vi "Experiment 23.vi"() -> ()   [LabVIEW 2026]
doc: "Experiment 23"
uses:
  <vilib>/AdvancedString/1D String Array to Delimited String (string).vi
  <vilib>/Analysis/baseanly.llb/Mean (DBL).vi
  <vilib>/Analysis/NI_AALBase.lvlib
panel:
  out "No. Of Iterations As Block Of Text (easy to copy into Excel)":string
  out "No. Of Iterations Executed - Loop 10":i32
  out "Output - Loop 10":dbl[](array[numeric]) format="%.3f"
  out "No. Of Iterations Executed - Loop 9":i32
  out "Output - Loop 9":dbl[](array[numeric]) format="%.3f"
  out "No. Of Iterations Executed - Loop 8":i32
  out "Output - Loop 8":dbl[](array[numeric]) format="%.3f"
  out "No. Of Iterations Executed - Loop 7":i32
  out "Output - Loop 7":dbl[](array[numeric]) format="%.3f"
  out "No. Of Iterations Executed - Loop 6":i32
  out "Output - Loop 6":dbl[](array[numeric]) format="%.3f"
  out "No. Of Iterations Executed - Loop 5":i32
  out "Output - Loop 5":dbl[](array[numeric]) format="%.3f"
  out "No. Of Iterations Executed - Loop 4":i32
  out "Output - Loop 4":dbl[](array[numeric]) format="%.3f"
  out "No. Of Iterations Executed - Loop 3":i32
  out "Output - Loop 3":dbl[](array[numeric]) format="%.3f"
  out "Avg. No. Of Iterations Executed - All Loops":dbl format="%.1f"
  out "No. Of Iterations Executed - Loop 2":i32
  out "Output - Loop 2":dbl[](array[numeric]) format="%.3f"
  out "No. Of Iterations Executed - Loop 1":i32
  out "Output - Loop 1":dbl[](array[numeric]) format="%.3f"
  out "Stop VI?":bool
  # "Experiment 23"
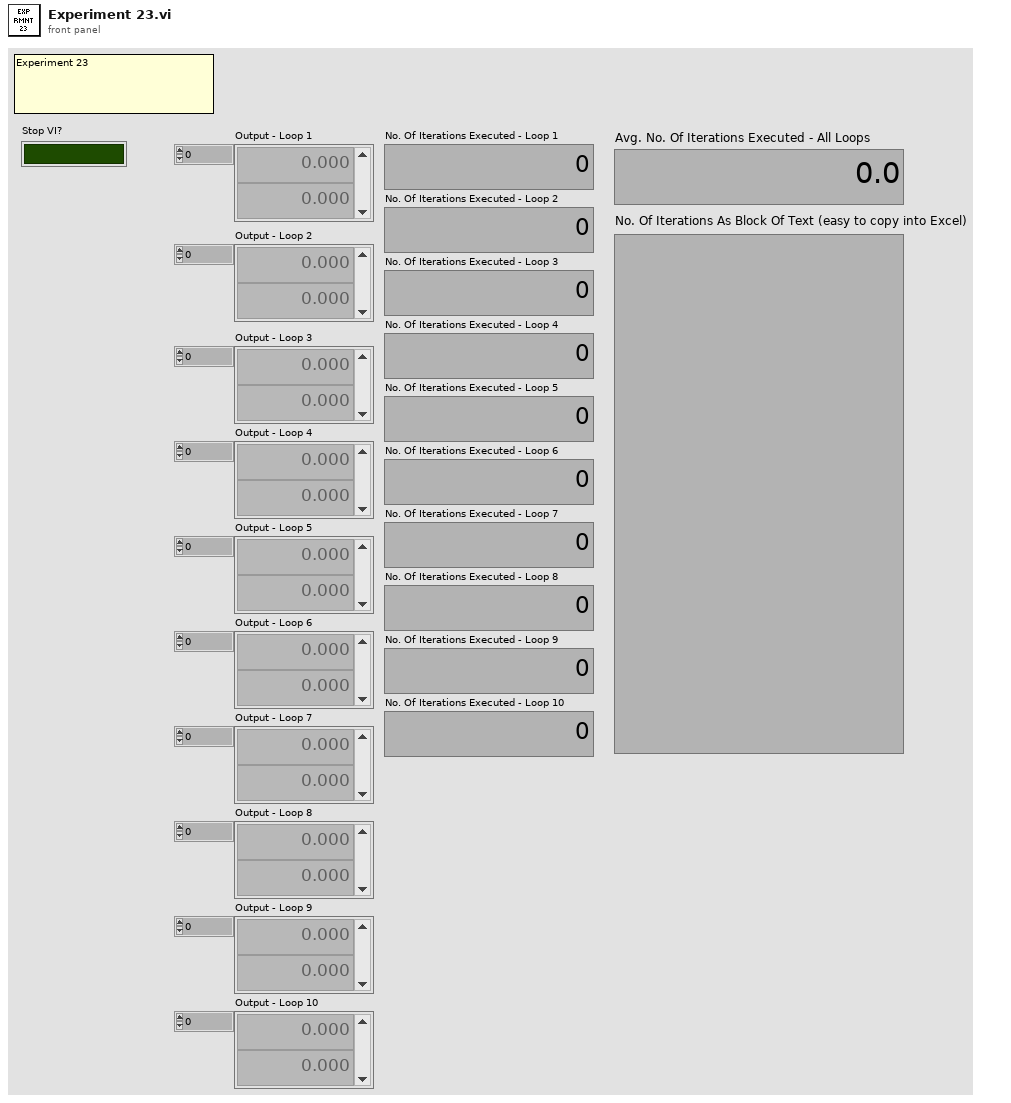
[diagram p1: front panel]
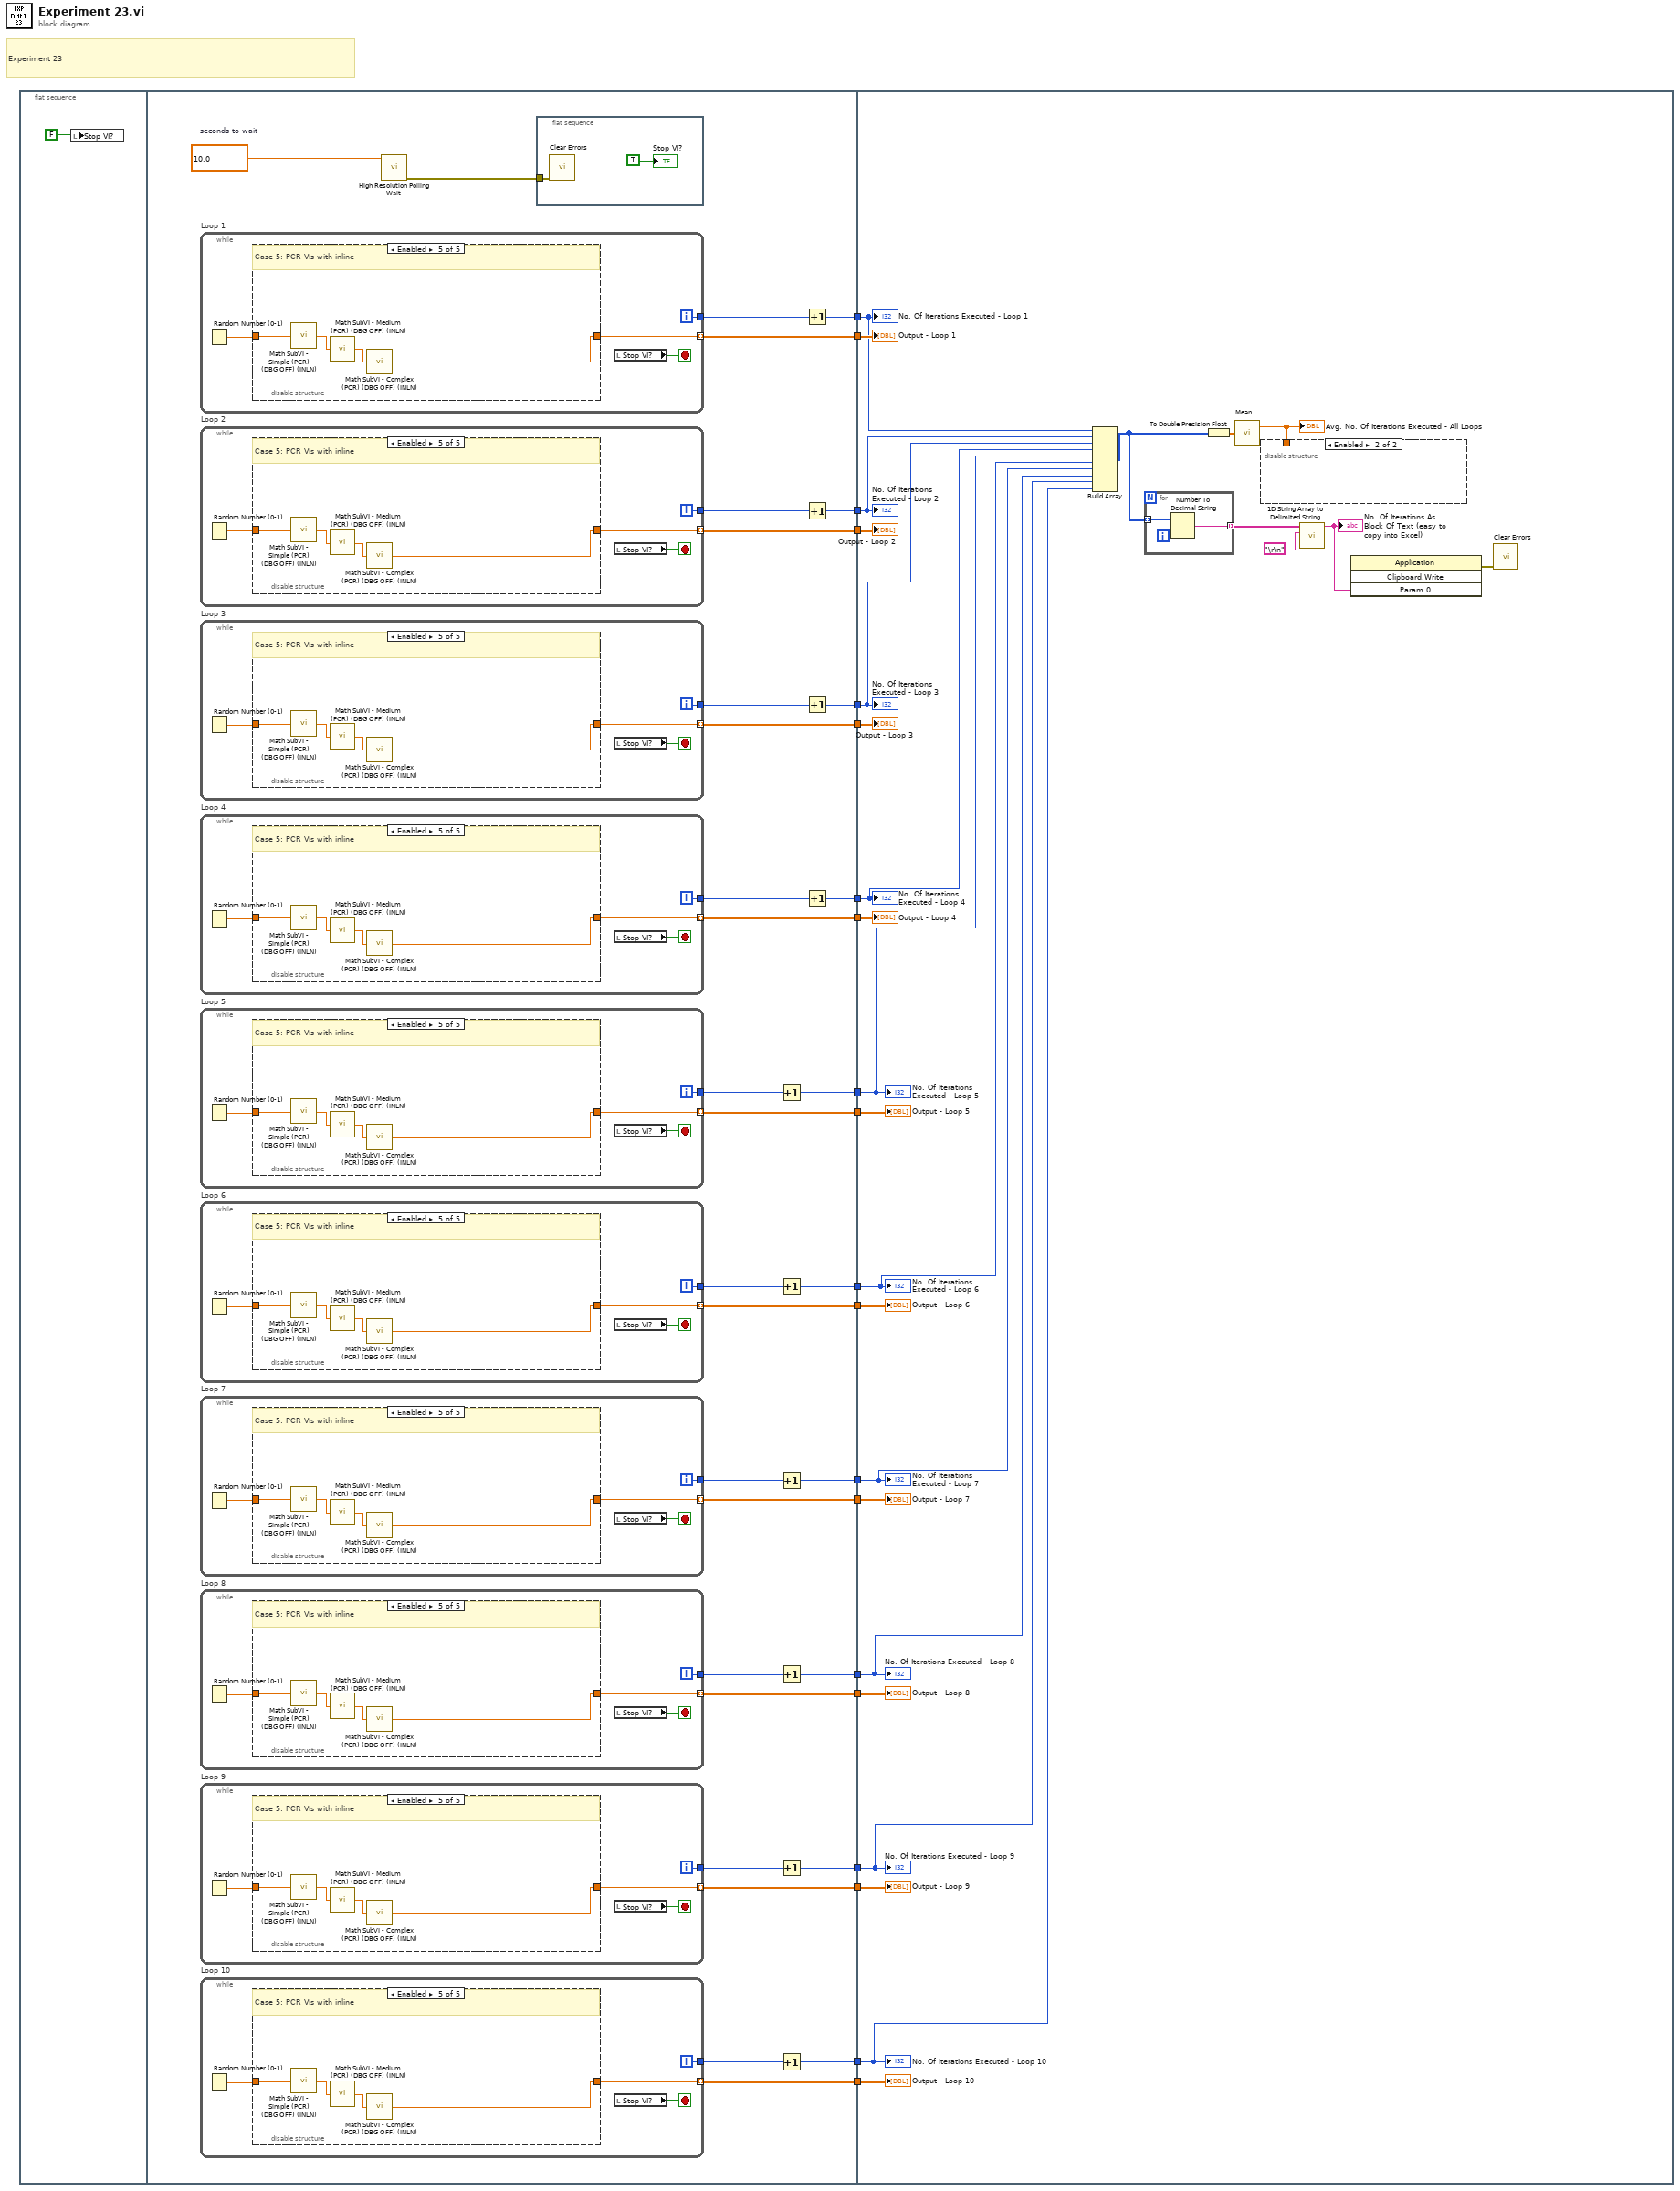
[diagram p0: block diagram]
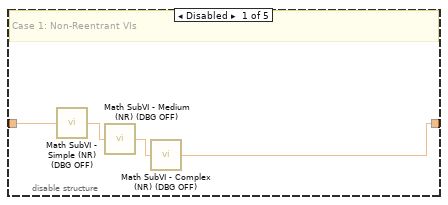
[diagram p2: hidden frame]
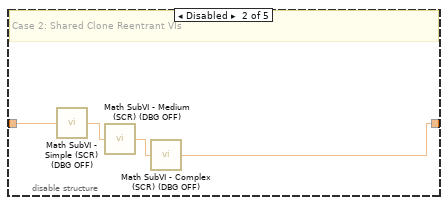
[diagram p3: hidden frame]
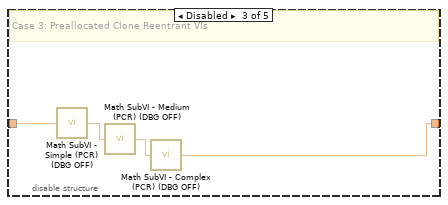
[diagram p4: hidden frame]
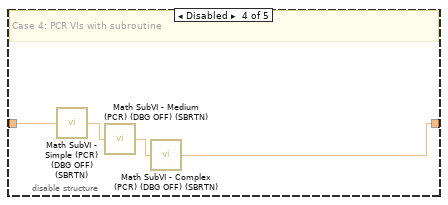
[diagram p5: hidden frame]
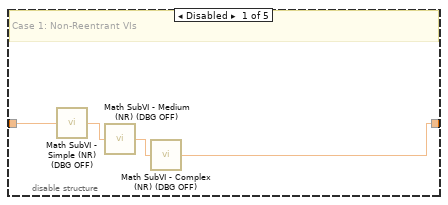
[diagram p6: hidden frame]
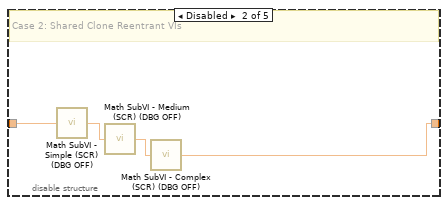
[diagram p7: hidden frame]
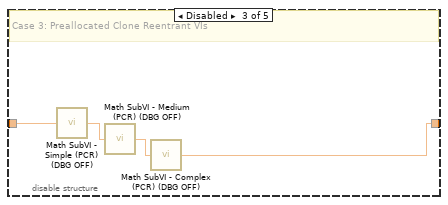
[diagram p8: hidden frame]
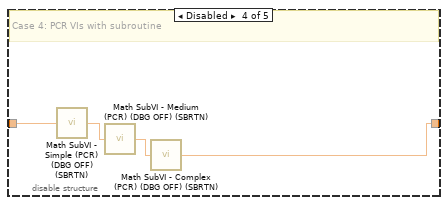
[diagram p9: hidden frame]
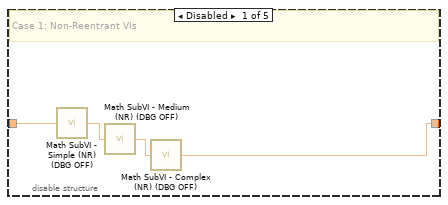
[diagram p10: hidden frame]
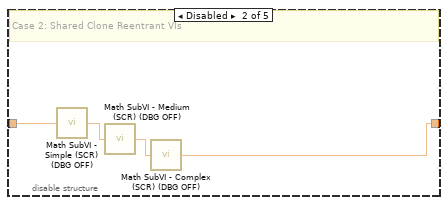
[diagram p11: hidden frame]
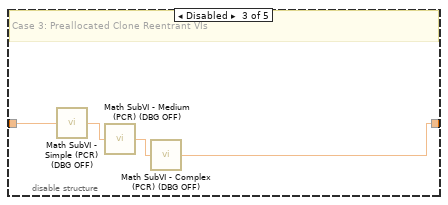
[diagram p12: hidden frame]
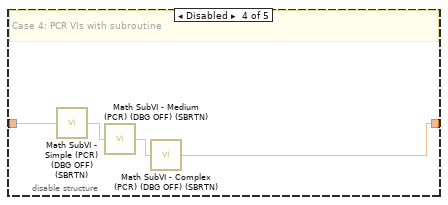
[diagram p13: hidden frame]
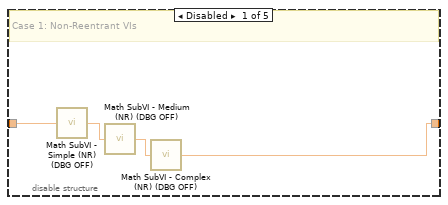
[diagram p14: hidden frame]
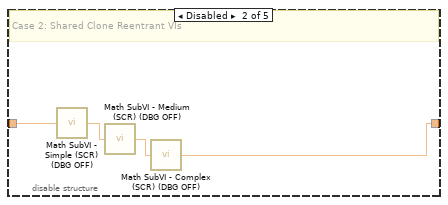
[diagram p15: hidden frame]
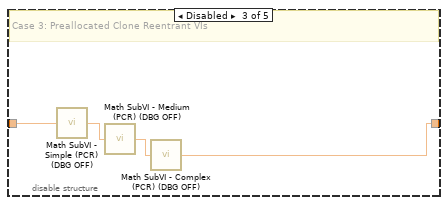
[diagram p16: hidden frame]
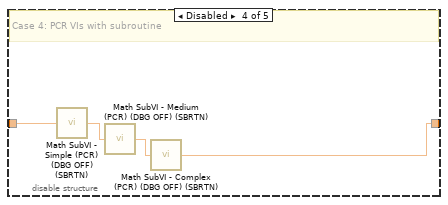
[diagram p17: hidden frame]
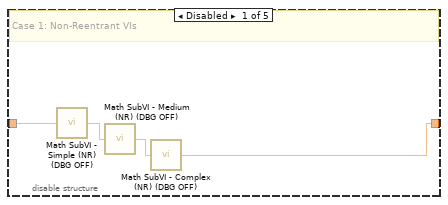
[diagram p18: hidden frame]
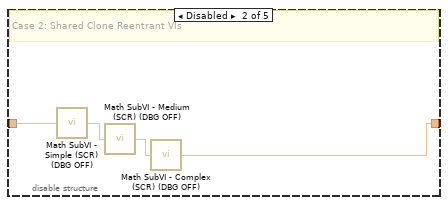
[diagram p19: hidden frame]
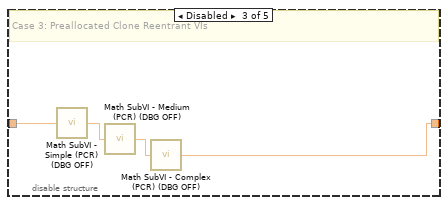
[diagram p20: hidden frame]
diagram:
  # "Experiment 23"
  n1 = flat-sequence {
    tunnel: [w51] -> w20
    tunnel: [w49] -> w19
    tunnel: [w48] -> w18
    tunnel: [w39] -> w17
    tunnel: [w47] -> w16
    tunnel: [w37] -> w15
    tunnel: [w35] -> w14
    tunnel: [w46] -> w13
    tunnel: [w33] -> w12
    tunnel: [w45] -> w11
    tunnel: [w31] -> w10
    tunnel: [w40] -> w9
    tunnel: [w29] -> w8
    tunnel: [w41] -> w7
    tunnel: [w27] -> w6
    tunnel: [w42] -> w5
    tunnel: [w25] -> w4
    tunnel: [w43] -> w3
    tunnel: [w22] -> w2
    tunnel: [w44] -> w1
    tunnel: w20 -> [w322]
    tunnel: w19 -> [w320]
    tunnel: w18 -> [w319]
    tunnel: w17 -> [w321]
    tunnel: w16 -> [w315]
    tunnel: w15 -> [w317]
    tunnel: w14 -> [w316]
    tunnel: w13 -> [w314]
    tunnel: w12 -> [w312]
    tunnel: w11 -> [w306]
    tunnel: w10 -> [w311]
    tunnel: w9 -> [w305]
    tunnel: w8 -> [w310]
    tunnel: w7 -> [w304]
    tunnel: w6 -> [w309]
    tunnel: w5 -> [w303]
    tunnel: w4 -> [w308]
    tunnel: w3 -> [w302]
    tunnel: w2 -> [w307]
    tunnel: w1 -> [w301]
    frame #0 {
      n2 = local write "Stop VI?"(FALSE) -> ()
    }
    frame #1 {
      w53 = 10.0  # seconds to wait
      n3 = while "Loop 1" {
        tunnel: [w271] -> w51 mode=indexing
        tunnel: [w272] -> w50
        i -> [w272]
        stop <- w273 stop-if-true
        n4 = Random Number (0-1)() -> (number: 0 to 1=w270:dbl)
        n5 = disable-structure shown="Enabled" {
          disable-tunnel: w270 -> [w277 w281 w285 w289 w293]
          disable-tunnel: [w276 w280 w284 w288 w292] -> w271
          frame Disabled {
            # "Case 1: Non-Reentrant VIs"
            n6 = call "Math SubVI - Simple (NR) (DBG OFF).vi"("Input"=w277) -> ("Output"=w274:dbl)
            n7 = call "Math SubVI - Medium (NR) (DBG OFF).vi"("Input"=w274) -> ("Output"=w275:dbl)
            n8 = call "Math SubVI - Complex (NR) (DBG OFF).vi"("Input"=w275) -> ("Output"=w276:dbl)
          }
          frame Disabled {
            # "Case 2: Shared Clone Reentrant VIs"
            n9 = call "Math SubVI - Simple (SCR) (DBG OFF).vi"("Input"=w281) -> ("Output"=w278:dbl)
            n10 = call "Math SubVI - Medium (SCR) (DBG OFF).vi"("Input"=w278) -> ("Output"=w279:dbl)
            n11 = call "Math SubVI - Complex (SCR) (DBG OFF).vi"("Input"=w279) -> ("Output"=w280:dbl)
          }
          frame Disabled {
            # "Case 3: Preallocated Clone Reentrant VIs"
            n12 = call "Math SubVI - Simple (PCR) (DBG OFF).vi"("Input"=w285) -> ("Output"=w282:dbl)
            n13 = call "Math SubVI - Medium (PCR) (DBG OFF).vi"("Input"=w282) -> ("Output"=w283:dbl)
            n14 = call "Math SubVI - Complex (PCR) (DBG OFF).vi"("Input"=w283) -> ("Output"=w284:dbl)
          }
          frame Disabled {
            # "Case 4: PCR VIs with subroutine"
            n15 = call "Math SubVI - Simple (PCR) (DBG OFF) (SBRTN).vi"("Input"=w289) -> ("Output"=w286:dbl)
            n16 = call "Math SubVI - Medium (PCR) (DBG OFF) (SBRTN).vi"("Input"=w286) -> ("Output"=w287:dbl)
            n17 = call "Math SubVI - Complex (PCR) (DBG OFF) (SBRTN).vi"("Input"=w287) -> ("Output"=w288:dbl)
          }
          frame Enabled {
            # "Case 5: PCR VIs with inline"
            n18 = call "Math SubVI - Simple (PCR) (DBG OFF) (INLN).vi"("Input"=w293) -> ("Output"=w290:dbl)
            n19 = call "Math SubVI - Medium (PCR) (DBG OFF) (INLN).vi"("Input"=w290) -> ("Output"=w291:dbl)
            n20 = call "Math SubVI - Complex (PCR) (DBG OFF) (INLN).vi"("Input"=w291) -> ("Output"=w292:dbl)
          }
        }
        n21 = local read "Stop VI?"() -> (w273:bool)
      }
      n22 = while "Loop 2" {
        tunnel: [w247] -> w39 mode=indexing
        tunnel: [w248] -> w38
        i -> [w248]
        stop <- w249 stop-if-true
        n23 = Random Number (0-1)() -> (number: 0 to 1=w246:dbl)
        n24 = disable-structure shown="Enabled" {
          disable-tunnel: w246 -> [w253 w257 w261 w265 w269]
          disable-tunnel: [w252 w256 w260 w264 w268] -> w247
          frame Disabled {
            # "Case 1: Non-Reentrant VIs"
            n25 = call "Math SubVI - Simple (NR) (DBG OFF).vi"("Input"=w253) -> ("Output"=w250:dbl)
            n26 = call "Math SubVI - Medium (NR) (DBG OFF).vi"("Input"=w250) -> ("Output"=w251:dbl)
            n27 = call "Math SubVI - Complex (NR) (DBG OFF).vi"("Input"=w251) -> ("Output"=w252:dbl)
          }
          frame Disabled {
            # "Case 2: Shared Clone Reentrant VIs"
            n28 = call "Math SubVI - Simple (SCR) (DBG OFF).vi"("Input"=w257) -> ("Output"=w254:dbl)
            n29 = call "Math SubVI - Medium (SCR) (DBG OFF).vi"("Input"=w254) -> ("Output"=w255:dbl)
            n30 = call "Math SubVI - Complex (SCR) (DBG OFF).vi"("Input"=w255) -> ("Output"=w256:dbl)
          }
          frame Disabled {
            # "Case 3: Preallocated Clone Reentrant VIs"
            n31 = call "Math SubVI - Simple (PCR) (DBG OFF).vi"("Input"=w261) -> ("Output"=w258:dbl)
            n32 = call "Math SubVI - Medium (PCR) (DBG OFF).vi"("Input"=w258) -> ("Output"=w259:dbl)
            n33 = call "Math SubVI - Complex (PCR) (DBG OFF).vi"("Input"=w259) -> ("Output"=w260:dbl)
          }
          frame Disabled {
            # "Case 4: PCR VIs with subroutine"
            n34 = call "Math SubVI - Simple (PCR) (DBG OFF) (SBRTN).vi"("Input"=w265) -> ("Output"=w262:dbl)
            n35 = call "Math SubVI - Medium (PCR) (DBG OFF) (SBRTN).vi"("Input"=w262) -> ("Output"=w263:dbl)
            n36 = call "Math SubVI - Complex (PCR) (DBG OFF) (SBRTN).vi"("Input"=w263) -> ("Output"=w264:dbl)
          }
          frame Enabled {
            # "Case 5: PCR VIs with inline"
            n37 = call "Math SubVI - Simple (PCR) (DBG OFF) (INLN).vi"("Input"=w269) -> ("Output"=w266:dbl)
            n38 = call "Math SubVI - Medium (PCR) (DBG OFF) (INLN).vi"("Input"=w266) -> ("Output"=w267:dbl)
            n39 = call "Math SubVI - Complex (PCR) (DBG OFF) (INLN).vi"("Input"=w267) -> ("Output"=w268:dbl)
          }
        }
        n40 = local read "Stop VI?"() -> (w249:bool)
      }
      n41 = while "Loop 3" {
        tunnel: [w223] -> w37 mode=indexing
        tunnel: [w224] -> w36
        i -> [w224]
        stop <- w225 stop-if-true
        n42 = Random Number (0-1)() -> (number: 0 to 1=w222:dbl)
        n43 = disable-structure shown="Enabled" {
          disable-tunnel: w222 -> [w229 w233 w237 w241 w245]
          disable-tunnel: [w228 w232 w236 w240 w244] -> w223
          frame Disabled {
            # "Case 1: Non-Reentrant VIs"
            n44 = call "Math SubVI - Simple (NR) (DBG OFF).vi"("Input"=w229) -> ("Output"=w226:dbl)
            n45 = call "Math SubVI - Medium (NR) (DBG OFF).vi"("Input"=w226) -> ("Output"=w227:dbl)
            n46 = call "Math SubVI - Complex (NR) (DBG OFF).vi"("Input"=w227) -> ("Output"=w228:dbl)
          }
          frame Disabled {
            # "Case 2: Shared Clone Reentrant VIs"
            n47 = call "Math SubVI - Simple (SCR) (DBG OFF).vi"("Input"=w233) -> ("Output"=w230:dbl)
            n48 = call "Math SubVI - Medium (SCR) (DBG OFF).vi"("Input"=w230) -> ("Output"=w231:dbl)
            n49 = call "Math SubVI - Complex (SCR) (DBG OFF).vi"("Input"=w231) -> ("Output"=w232:dbl)
          }
          frame Disabled {
            # "Case 3: Preallocated Clone Reentrant VIs"
            n50 = call "Math SubVI - Simple (PCR) (DBG OFF).vi"("Input"=w237) -> ("Output"=w234:dbl)
            n51 = call "Math SubVI - Medium (PCR) (DBG OFF).vi"("Input"=w234) -> ("Output"=w235:dbl)
            n52 = call "Math SubVI - Complex (PCR) (DBG OFF).vi"("Input"=w235) -> ("Output"=w236:dbl)
          }
          frame Disabled {
            # "Case 4: PCR VIs with subroutine"
            n53 = call "Math SubVI - Simple (PCR) (DBG OFF) (SBRTN).vi"("Input"=w241) -> ("Output"=w238:dbl)
            n54 = call "Math SubVI - Medium (PCR) (DBG OFF) (SBRTN).vi"("Input"=w238) -> ("Output"=w239:dbl)
            n55 = call "Math SubVI - Complex (PCR) (DBG OFF) (SBRTN).vi"("Input"=w239) -> ("Output"=w240:dbl)
          }
          frame Enabled {
            # "Case 5: PCR VIs with inline"
            n56 = call "Math SubVI - Simple (PCR) (DBG OFF) (INLN).vi"("Input"=w245) -> ("Output"=w242:dbl)
            n57 = call "Math SubVI - Medium (PCR) (DBG OFF) (INLN).vi"("Input"=w242) -> ("Output"=w243:dbl)
            n58 = call "Math SubVI - Complex (PCR) (DBG OFF) (INLN).vi"("Input"=w243) -> ("Output"=w244:dbl)
          }
        }
        n59 = local read "Stop VI?"() -> (w225:bool)
      }
      n60 = while "Loop 4" {
        tunnel: [w199] -> w35 mode=indexing
        tunnel: [w200] -> w34
        i -> [w200]
        stop <- w201 stop-if-true
        n61 = Random Number (0-1)() -> (number: 0 to 1=w198:dbl)
        n62 = disable-structure shown="Enabled" {
          disable-tunnel: w198 -> [w205 w209 w213 w217 w221]
          disable-tunnel: [w204 w208 w212 w216 w220] -> w199
          frame Disabled {
            # "Case 1: Non-Reentrant VIs"
            n63 = call "Math SubVI - Simple (NR) (DBG OFF).vi"("Input"=w205) -> ("Output"=w202:dbl)
            n64 = call "Math SubVI - Medium (NR) (DBG OFF).vi"("Input"=w202) -> ("Output"=w203:dbl)
            n65 = call "Math SubVI - Complex (NR) (DBG OFF).vi"("Input"=w203) -> ("Output"=w204:dbl)
          }
          frame Disabled {
            # "Case 2: Shared Clone Reentrant VIs"
            n66 = call "Math SubVI - Simple (SCR) (DBG OFF).vi"("Input"=w209) -> ("Output"=w206:dbl)
            n67 = call "Math SubVI - Medium (SCR) (DBG OFF).vi"("Input"=w206) -> ("Output"=w207:dbl)
            n68 = call "Math SubVI - Complex (SCR) (DBG OFF).vi"("Input"=w207) -> ("Output"=w208:dbl)
          }
          frame Disabled {
            # "Case 3: Preallocated Clone Reentrant VIs"
            n69 = call "Math SubVI - Simple (PCR) (DBG OFF).vi"("Input"=w213) -> ("Output"=w210:dbl)
            n70 = call "Math SubVI - Medium (PCR) (DBG OFF).vi"("Input"=w210) -> ("Output"=w211:dbl)
            n71 = call "Math SubVI - Complex (PCR) (DBG OFF).vi"("Input"=w211) -> ("Output"=w212:dbl)
          }
          frame Disabled {
            # "Case 4: PCR VIs with subroutine"
            n72 = call "Math SubVI - Simple (PCR) (DBG OFF) (SBRTN).vi"("Input"=w217) -> ("Output"=w214:dbl)
            n73 = call "Math SubVI - Medium (PCR) (DBG OFF) (SBRTN).vi"("Input"=w214) -> ("Output"=w215:dbl)
            n74 = call "Math SubVI - Complex (PCR) (DBG OFF) (SBRTN).vi"("Input"=w215) -> ("Output"=w216:dbl)
          }
          frame Enabled {
            # "Case 5: PCR VIs with inline"
            n75 = call "Math SubVI - Simple (PCR) (DBG OFF) (INLN).vi"("Input"=w221) -> ("Output"=w218:dbl)
            n76 = call "Math SubVI - Medium (PCR) (DBG OFF) (INLN).vi"("Input"=w218) -> ("Output"=w219:dbl)
            n77 = call "Math SubVI - Complex (PCR) (DBG OFF) (INLN).vi"("Input"=w219) -> ("Output"=w220:dbl)
          }
        }
        n78 = local read "Stop VI?"() -> (w201:bool)
      }
      n79 = while "Loop 5" {
        tunnel: [w175] -> w33 mode=indexing
        tunnel: [w176] -> w32
        i -> [w176]
        stop <- w177 stop-if-true
        n80 = Random Number (0-1)() -> (number: 0 to 1=w174:dbl)
        n81 = disable-structure shown="Enabled" {
          disable-tunnel: w174 -> [w181 w185 w189 w193 w197]
          disable-tunnel: [w180 w184 w188 w192 w196] -> w175
          frame Disabled {
            # "Case 1: Non-Reentrant VIs"
            n82 = call "Math SubVI - Simple (NR) (DBG OFF).vi"("Input"=w181) -> ("Output"=w178:dbl)
            n83 = call "Math SubVI - Medium (NR) (DBG OFF).vi"("Input"=w178) -> ("Output"=w179:dbl)
            n84 = call "Math SubVI - Complex (NR) (DBG OFF).vi"("Input"=w179) -> ("Output"=w180:dbl)
          }
          frame Disabled {
            # "Case 2: Shared Clone Reentrant VIs"
            n85 = call "Math SubVI - Simple (SCR) (DBG OFF).vi"("Input"=w185) -> ("Output"=w182:dbl)
            n86 = call "Math SubVI - Medium (SCR) (DBG OFF).vi"("Input"=w182) -> ("Output"=w183:dbl)
            n87 = call "Math SubVI - Complex (SCR) (DBG OFF).vi"("Input"=w183) -> ("Output"=w184:dbl)
          }
          frame Disabled {
            # "Case 3: Preallocated Clone Reentrant VIs"
            n88 = call "Math SubVI - Simple (PCR) (DBG OFF).vi"("Input"=w189) -> ("Output"=w186:dbl)
            n89 = call "Math SubVI - Medium (PCR) (DBG OFF).vi"("Input"=w186) -> ("Output"=w187:dbl)
            n90 = call "Math SubVI - Complex (PCR) (DBG OFF).vi"("Input"=w187) -> ("Output"=w188:dbl)
          }
          frame Disabled {
            # "Case 4: PCR VIs with subroutine"
            n91 = call "Math SubVI - Simple (PCR) (DBG OFF) (SBRTN).vi"("Input"=w193) -> ("Output"=w190:dbl)
            n92 = call "Math SubVI - Medium (PCR) (DBG OFF) (SBRTN).vi"("Input"=w190) -> ("Output"=w191:dbl)
            n93 = call "Math SubVI - Complex (PCR) (DBG OFF) (SBRTN).vi"("Input"=w191) -> ("Output"=w192:dbl)
          }
          frame Enabled {
            # "Case 5: PCR VIs with inline"
            n94 = call "Math SubVI - Simple (PCR) (DBG OFF) (INLN).vi"("Input"=w197) -> ("Output"=w194:dbl)
            n95 = call "Math SubVI - Medium (PCR) (DBG OFF) (INLN).vi"("Input"=w194) -> ("Output"=w195:dbl)
            n96 = call "Math SubVI - Complex (PCR) (DBG OFF) (INLN).vi"("Input"=w195) -> ("Output"=w196:dbl)
          }
        }
        n97 = local read "Stop VI?"() -> (w177:bool)
      }
      n98 = while "Loop 6" {
        tunnel: [w151] -> w31 mode=indexing
        tunnel: [w152] -> w30
        i -> [w152]
        stop <- w153 stop-if-true
        n99 = Random Number (0-1)() -> (number: 0 to 1=w150:dbl)
        n100 = disable-structure shown="Enabled" {
          disable-tunnel: w150 -> [w157 w161 w165 w169 w173]
          disable-tunnel: [w156 w160 w164 w168 w172] -> w151
          frame Disabled {
            # "Case 1: Non-Reentrant VIs"
            n101 = call "Math SubVI - Simple (NR) (DBG OFF).vi"("Input"=w157) -> ("Output"=w154:dbl)
            n102 = call "Math SubVI - Medium (NR) (DBG OFF).vi"("Input"=w154) -> ("Output"=w155:dbl)
            n103 = call "Math SubVI - Complex (NR) (DBG OFF).vi"("Input"=w155) -> ("Output"=w156:dbl)
          }
          frame Disabled {
            # "Case 2: Shared Clone Reentrant VIs"
            n104 = call "Math SubVI - Simple (SCR) (DBG OFF).vi"("Input"=w161) -> ("Output"=w158:dbl)
            n105 = call "Math SubVI - Medium (SCR) (DBG OFF).vi"("Input"=w158) -> ("Output"=w159:dbl)
            n106 = call "Math SubVI - Complex (SCR) (DBG OFF).vi"("Input"=w159) -> ("Output"=w160:dbl)
          }
          frame Disabled {
            # "Case 3: Preallocated Clone Reentrant VIs"
            n107 = call "Math SubVI - Simple (PCR) (DBG OFF).vi"("Input"=w165) -> ("Output"=w162:dbl)
            n108 = call "Math SubVI - Medium (PCR) (DBG OFF).vi"("Input"=w162) -> ("Output"=w163:dbl)
            n109 = call "Math SubVI - Complex (PCR) (DBG OFF).vi"("Input"=w163) -> ("Output"=w164:dbl)
          }
          frame Disabled {
            # "Case 4: PCR VIs with subroutine"
            n110 = call "Math SubVI - Simple (PCR) (DBG OFF) (SBRTN).vi"("Input"=w169) -> ("Output"=w166:dbl)
            n111 = call "Math SubVI - Medium (PCR) (DBG OFF) (SBRTN).vi"("Input"=w166) -> ("Output"=w167:dbl)
            n112 = call "Math SubVI - Complex (PCR) (DBG OFF) (SBRTN).vi"("Input"=w167) -> ("Output"=w168:dbl)
          }
          frame Enabled {
            # "Case 5: PCR VIs with inline"
            n113 = call "Math SubVI - Simple (PCR) (DBG OFF) (INLN).vi"("Input"=w173) -> ("Output"=w170:dbl)
            n114 = call "Math SubVI - Medium (PCR) (DBG OFF) (INLN).vi"("Input"=w170) -> ("Output"=w171:dbl)
            n115 = call "Math SubVI - Complex (PCR) (DBG OFF) (INLN).vi"("Input"=w171) -> ("Output"=w172:dbl)
          }
        }
        n116 = local read "Stop VI?"() -> (w153:bool)
      }
      n117 = while "Loop 7" {
        tunnel: [w127] -> w29 mode=indexing
        tunnel: [w128] -> w28
        i -> [w128]
        stop <- w129 stop-if-true
        n118 = Random Number (0-1)() -> (number: 0 to 1=w126:dbl)
        n119 = disable-structure shown="Enabled" {
          disable-tunnel: w126 -> [w133 w137 w141 w145 w149]
          disable-tunnel: [w132 w136 w140 w144 w148] -> w127
          frame Disabled {
            # "Case 1: Non-Reentrant VIs"
            n120 = call "Math SubVI - Simple (NR) (DBG OFF).vi"("Input"=w133) -> ("Output"=w130:dbl)
            n121 = call "Math SubVI - Medium (NR) (DBG OFF).vi"("Input"=w130) -> ("Output"=w131:dbl)
            n122 = call "Math SubVI - Complex (NR) (DBG OFF).vi"("Input"=w131) -> ("Output"=w132:dbl)
          }
          frame Disabled {
            # "Case 2: Shared Clone Reentrant VIs"
            n123 = call "Math SubVI - Simple (SCR) (DBG OFF).vi"("Input"=w137) -> ("Output"=w134:dbl)
            n124 = call "Math SubVI - Medium (SCR) (DBG OFF).vi"("Input"=w134) -> ("Output"=w135:dbl)
            n125 = call "Math SubVI - Complex (SCR) (DBG OFF).vi"("Input"=w135) -> ("Output"=w136:dbl)
          }
          frame Disabled {
            # "Case 3: Preallocated Clone Reentrant VIs"
            n126 = call "Math SubVI - Simple (PCR) (DBG OFF).vi"("Input"=w141) -> ("Output"=w138:dbl)
            n127 = call "Math SubVI - Medium (PCR) (DBG OFF).vi"("Input"=w138) -> ("Output"=w139:dbl)
            n128 = call "Math SubVI - Complex (PCR) (DBG OFF).vi"("Input"=w139) -> ("Output"=w140:dbl)
          }
          frame Disabled {
            # "Case 4: PCR VIs with subroutine"
            n129 = call "Math SubVI - Simple (PCR) (DBG OFF) (SBRTN).vi"("Input"=w145) -> ("Output"=w142:dbl)
            n130 = call "Math SubVI - Medium (PCR) (DBG OFF) (SBRTN).vi"("Input"=w142) -> ("Output"=w143:dbl)
            n131 = call "Math SubVI - Complex (PCR) (DBG OFF) (SBRTN).vi"("Input"=w143) -> ("Output"=w144:dbl)
          }
          frame Enabled {
            # "Case 5: PCR VIs with inline"
            n132 = call "Math SubVI - Simple (PCR) (DBG OFF) (INLN).vi"("Input"=w149) -> ("Output"=w146:dbl)
            n133 = call "Math SubVI - Medium (PCR) (DBG OFF) (INLN).vi"("Input"=w146) -> ("Output"=w147:dbl)
            n134 = call "Math SubVI - Complex (PCR) (DBG OFF) (INLN).vi"("Input"=w147) -> ("Output"=w148:dbl)
          }
        }
        n135 = local read "Stop VI?"() -> (w129:bool)
      }
      n136 = while "Loop 8" {
        tunnel: [w103] -> w27 mode=indexing
        tunnel: [w104] -> w26
        i -> [w104]
        stop <- w105 stop-if-true
        n137 = Random Number (0-1)() -> (number: 0 to 1=w102:dbl)
        n138 = disable-structure shown="Enabled" {
          disable-tunnel: w102 -> [w109 w113 w117 w121 w125]
          disable-tunnel: [w108 w112 w116 w120 w124] -> w103
          frame Disabled {
            # "Case 1: Non-Reentrant VIs"
            n139 = call "Math SubVI - Simple (NR) (DBG OFF).vi"("Input"=w109) -> ("Output"=w106:dbl)
            n140 = call "Math SubVI - Medium (NR) (DBG OFF).vi"("Input"=w106) -> ("Output"=w107:dbl)
            n141 = call "Math SubVI - Complex (NR) (DBG OFF).vi"("Input"=w107) -> ("Output"=w108:dbl)
          }
          frame Disabled {
            # "Case 2: Shared Clone Reentrant VIs"
            n142 = call "Math SubVI - Simple (SCR) (DBG OFF).vi"("Input"=w113) -> ("Output"=w110:dbl)
            n143 = call "Math SubVI - Medium (SCR) (DBG OFF).vi"("Input"=w110) -> ("Output"=w111:dbl)
            n144 = call "Math SubVI - Complex (SCR) (DBG OFF).vi"("Input"=w111) -> ("Output"=w112:dbl)
          }
          frame Disabled {
            # "Case 3: Preallocated Clone Reentrant VIs"
            n145 = call "Math SubVI - Simple (PCR) (DBG OFF).vi"("Input"=w117) -> ("Output"=w114:dbl)
            n146 = call "Math SubVI - Medium (PCR) (DBG OFF).vi"("Input"=w114) -> ("Output"=w115:dbl)
            n147 = call "Math SubVI - Complex (PCR) (DBG OFF).vi"("Input"=w115) -> ("Output"=w116:dbl)
          }
          frame Disabled {
            # "Case 4: PCR VIs with subroutine"
            n148 = call "Math SubVI - Simple (PCR) (DBG OFF) (SBRTN).vi"("Input"=w121) -> ("Output"=w118:dbl)
            n149 = call "Math SubVI - Medium (PCR) (DBG OFF) (SBRTN).vi"("Input"=w118) -> ("Output"=w119:dbl)
            n150 = call "Math SubVI - Complex (PCR) (DBG OFF) (SBRTN).vi"("Input"=w119) -> ("Output"=w120:dbl)
          }
          frame Enabled {
            # "Case 5: PCR VIs with inline"
            n151 = call "Math SubVI - Simple (PCR) (DBG OFF) (INLN).vi"("Input"=w125) -> ("Output"=w122:dbl)
            n152 = call "Math SubVI - Medium (PCR) (DBG OFF) (INLN).vi"("Input"=w122) -> ("Output"=w123:dbl)
            n153 = call "Math SubVI - Complex (PCR) (DBG OFF) (INLN).vi"("Input"=w123) -> ("Output"=w124:dbl)
          }
        }
        n154 = local read "Stop VI?"() -> (w105:bool)
      }
      n155 = while "Loop 9" {
        tunnel: [w79] -> w25 mode=indexing
        tunnel: [w80] -> w24
        i -> [w80]
        stop <- w81 stop-if-true
        n156 = Random Number (0-1)() -> (number: 0 to 1=w78:dbl)
        n157 = disable-structure shown="Enabled" {
          disable-tunnel: w78 -> [w85 w89 w93 w97 w101]
          disable-tunnel: [w84 w88 w92 w96 w100] -> w79
          frame Disabled {
            # "Case 1: Non-Reentrant VIs"
            n158 = call "Math SubVI - Simple (NR) (DBG OFF).vi"("Input"=w85) -> ("Output"=w82:dbl)
            n159 = call "Math SubVI - Medium (NR) (DBG OFF).vi"("Input"=w82) -> ("Output"=w83:dbl)
            n160 = call "Math SubVI - Complex (NR) (DBG OFF).vi"("Input"=w83) -> ("Output"=w84:dbl)
          }
          frame Disabled {
            # "Case 2: Shared Clone Reentrant VIs"
            n161 = call "Math SubVI - Simple (SCR) (DBG OFF).vi"("Input"=w89) -> ("Output"=w86:dbl)
            n162 = call "Math SubVI - Medium (SCR) (DBG OFF).vi"("Input"=w86) -> ("Output"=w87:dbl)
            n163 = call "Math SubVI - Complex (SCR) (DBG OFF).vi"("Input"=w87) -> ("Output"=w88:dbl)
          }
          frame Disabled {
            # "Case 3: Preallocated Clone Reentrant VIs"
            n164 = call "Math SubVI - Simple (PCR) (DBG OFF).vi"("Input"=w93) -> ("Output"=w90:dbl)
            n165 = call "Math SubVI - Medium (PCR) (DBG OFF).vi"("Input"=w90) -> ("Output"=w91:dbl)
            n166 = call "Math SubVI - Complex (PCR) (DBG OFF).vi"("Input"=w91) -> ("Output"=w92:dbl)
          }
          frame Disabled {
            # "Case 4: PCR VIs with subroutine"
            n167 = call "Math SubVI - Simple (PCR) (DBG OFF) (SBRTN).vi"("Input"=w97) -> ("Output"=w94:dbl)
            n168 = call "Math SubVI - Medium (PCR) (DBG OFF) (SBRTN).vi"("Input"=w94) -> ("Output"=w95:dbl)
            n169 = call "Math SubVI - Complex (PCR) (DBG OFF) (SBRTN).vi"("Input"=w95) -> ("Output"=w96:dbl)
          }
          frame Enabled {
            # "Case 5: PCR VIs with inline"
            n170 = call "Math SubVI - Simple (PCR) (DBG OFF) (INLN).vi"("Input"=w101) -> ("Output"=w98:dbl)
            n171 = call "Math SubVI - Medium (PCR) (DBG OFF) (INLN).vi"("Input"=w98) -> ("Output"=w99:dbl)
            n172 = call "Math SubVI - Complex (PCR) (DBG OFF) (INLN).vi"("Input"=w99) -> ("Output"=w100:dbl)
          }
        }
        n173 = local read "Stop VI?"() -> (w81:bool)
      }
      n174 = while "Loop 10" {
        tunnel: [w55] -> w22 mode=indexing
        tunnel: [w56] -> w23
        i -> [w56]
        stop <- w57 stop-if-true
        n175 = Random Number (0-1)() -> (number: 0 to 1=w54:dbl)
        n176 = disable-structure shown="Enabled" {
          disable-tunnel: w54 -> [w61 w65 w69 w73 w77]
          disable-tunnel: [w60 w64 w68 w72 w76] -> w55
          frame Disabled {
            # "Case 1: Non-Reentrant VIs"
            n177 = call "Math SubVI - Simple (NR) (DBG OFF).vi"("Input"=w61) -> ("Output"=w58:dbl)
            n178 = call "Math SubVI - Medium (NR) (DBG OFF).vi"("Input"=w58) -> ("Output"=w59:dbl)
            n179 = call "Math SubVI - Complex (NR) (DBG OFF).vi"("Input"=w59) -> ("Output"=w60:dbl)
          }
          frame Disabled {
            # "Case 2: Shared Clone Reentrant VIs"
            n180 = call "Math SubVI - Simple (SCR) (DBG OFF).vi"("Input"=w65) -> ("Output"=w62:dbl)
            n181 = call "Math SubVI - Medium (SCR) (DBG OFF).vi"("Input"=w62) -> ("Output"=w63:dbl)
            n182 = call "Math SubVI - Complex (SCR) (DBG OFF).vi"("Input"=w63) -> ("Output"=w64:dbl)
          }
          frame Disabled {
            # "Case 3: Preallocated Clone Reentrant VIs"
            n183 = call "Math SubVI - Simple (PCR) (DBG OFF).vi"("Input"=w69) -> ("Output"=w66:dbl)
            n184 = call "Math SubVI - Medium (PCR) (DBG OFF).vi"("Input"=w66) -> ("Output"=w67:dbl)
            n185 = call "Math SubVI - Complex (PCR) (DBG OFF).vi"("Input"=w67) -> ("Output"=w68:dbl)
          }
          frame Disabled {
            # "Case 4: PCR VIs with subroutine"
            n186 = call "Math SubVI - Simple (PCR) (DBG OFF) (SBRTN).vi"("Input"=w73) -> ("Output"=w70:dbl)
            n187 = call "Math SubVI - Medium (PCR) (DBG OFF) (SBRTN).vi"("Input"=w70) -> ("Output"=w71:dbl)
            n188 = call "Math SubVI - Complex (PCR) (DBG OFF) (SBRTN).vi"("Input"=w71) -> ("Output"=w72:dbl)
          }
          frame Enabled {
            # "Case 5: PCR VIs with inline"
            n189 = call "Math SubVI - Simple (PCR) (DBG OFF) (INLN).vi"("Input"=w77) -> ("Output"=w74:dbl)
            n190 = call "Math SubVI - Medium (PCR) (DBG OFF) (INLN).vi"("Input"=w74) -> ("Output"=w75:dbl)
            n191 = call "Math SubVI - Complex (PCR) (DBG OFF) (INLN).vi"("Input"=w75) -> ("Output"=w76:dbl)
          }
        }
        n192 = local read "Stop VI?"() -> (w57:bool)
      }
      n193 = call <vilib>:"High Resolution Polling Wait.vi"("seconds to wait"=w53) -> ("error out"=w52:errorcluster)  [unwired: 10 in]
      n194 = flat-sequence {
        tunnel: w52 -> [w294]
        frame #0 {
          n195 = call <vilib>:"Clear Errors.vi"("error in (no error)"=w294) -> ()  [unwired: 5 in, 2 out]
          "Stop VI?" <- TRUE
        }
      }
      n196 = Increment(x=w32) -> (x+1=w45:i32)
      n197 = Increment(x=w30) -> (x+1=w40:i32)
      n198 = Increment(x=w28) -> (x+1=w41:i32)
      n199 = Increment(x=w26) -> (x+1=w42:i32)
      n200 = Increment(x=w24) -> (x+1=w43:i32)
      n201 = Increment(x=w23) -> (x+1=w44:i32)
      n202 = Increment(x=w50) -> (x+1=w49:i32)
      n203 = Increment(x=w38) -> (x+1=w48:i32)
      n204 = Increment(x=w36) -> (x+1=w47:i32)
      n205 = Increment(x=w34) -> (x+1=w46:i32)
    }
    frame #2 {
      n206 = Build Array(w320, w319, w315, w314, w306, w305, w304, w303, w302, w301) -> (w300:i32[])
      n207 = for {
        tunnel: w300 -> [w326] mode=indexing
        tunnel: [w325] -> w299 mode=indexing
        n208 = Number To Decimal String(number=w326) -> (decimal integer string=w325:string)  [unwired: 1 in]
      }
      n209 = To Double Precision Float(number=w300) -> (double precision float=w313:dbl[])
      n210 = call-poly <vilib>:"Mean.vi"("X"=w313) -> ("mean"=w318:dbl)  [unwired: 1 out]
      "Avg. No. Of Iterations Executed - All Loops" <- w318
      n211 = disable-structure shown="Enabled" {
        disable-tunnel: w318 -> [w324 _]
        frame Disabled {
          n212 = call "Copy Result To Clipboard.vi"("No. Of Decimal Places (6)"=u32 1, "Input"=w324) -> ()
        }
        frame Enabled {
        }
      }
      n213 = call-poly <vilib>:"1D String Array to Delimited String.vi"("delimiter"="\r\n", "string array"=w299) -> ("delimited string"=w296:string)  [unwired: 9 in]
      "No. Of Iterations As Block Of Text (easy to copy into Excel)" <- w296
      n214 = invoke class="Application" method="Clipboard.Write"("Param 0"=w296) -> (error out=w297:errorcluster)  [unwired: 3 in, 3 out]
      n215 = call <vilib>:"Clear Errors.vi"("error in (no error)"=w297) -> ()  [unwired: 5 in, 2 out]
      "No. Of Iterations Executed - Loop 1" <- w320
      "Output - Loop 1" <- w322
      "No. Of Iterations Executed - Loop 2" <- w319
      "Output - Loop 2" <- w321
      "No. Of Iterations Executed - Loop 3" <- w315
      "Output - Loop 3" <- w317
      "No. Of Iterations Executed - Loop 4" <- w314
      "Output - Loop 4" <- w316
      "No. Of Iterations Executed - Loop 5" <- w306
      "Output - Loop 5" <- w312
      "No. Of Iterations Executed - Loop 6" <- w305
      "Output - Loop 6" <- w311
      "No. Of Iterations Executed - Loop 7" <- w304
      "Output - Loop 7" <- w310
      "No. Of Iterations Executed - Loop 8" <- w303
      "Output - Loop 8" <- w309
      "No. Of Iterations Executed - Loop 9" <- w302
      "Output - Loop 9" <- w308
      "No. Of Iterations Executed - Loop 10" <- w301
      "Output - Loop 10" <- w307
    }
  }
